vi "MDAQ_ReverseCalibration.vi"(8 "MDU Velocity":dbl, 9 "MDAQ Calibration":dbl, 10 "Main Cluster in":T1, 11 "Status_Cluster In":T2 {"GATESTOP" format="%04x"; "GATESTRT" format="%04x"; "AMPLITUDE" format="%04x"; "M_CYCLES" format="%04x"; "N_CYCLES" format="%04x"; "STEP" format="%04x"; "BASE" format="%04x"; "CHAN" format="%04x"}) -> (1 "Scaler":dbl, 2 "output cluster":T1)   [LabVIEW 2021]
uses:
  <vilib>/Analysis/NI_AALPro.lvlib
  Status_Cluster.ctl
  GUI_Def.ctl
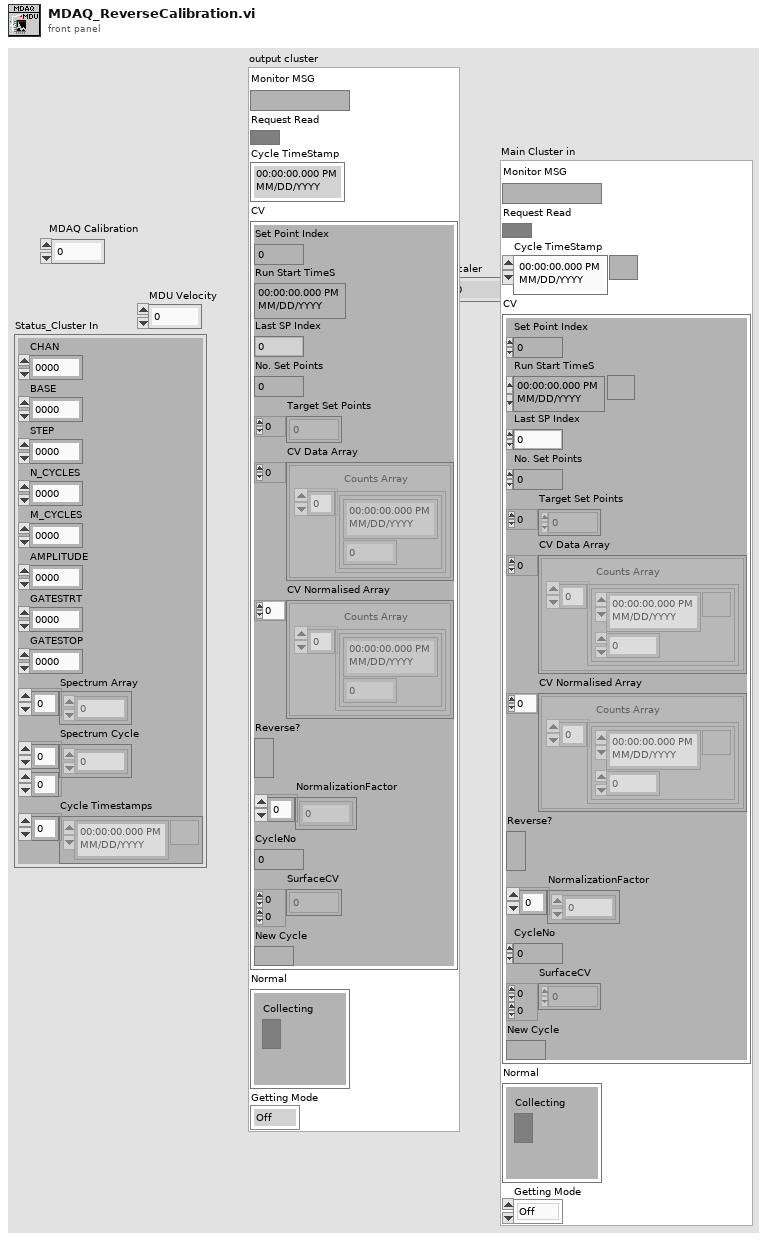
[diagram p1: front panel]
types:
  T1 = typedef "GUI_Def.ctl" = cluster{"Monitor MSG":string, "Request Read":bool, "Cycle TimeStamp":timestamp, "CV":cluster{"Set Point Index":u32, "Run Start TimeS":timestamp, "Last SP Index":u32, "No. Set Points":u32, "Target Set Points":dbl[], "CV Data Array":cluster{"Counts Array":cluster{timestamp, i32}[]}[], "CV Normalised Array":cluster{"Counts Array":cluster{timestamp, dbl}[]}[], "Reverse?":bool, "NormalizationFactor":i32[], "CycleNo":i32, "SurfaceCV":dbl[][], "New Cycle":bool}, "Normal":cluster{"Collecting":bool}, "Getting Mode":enum16{"Off", "Normal", "CV"}}
  T2 = typedef "Status_Cluster.ctl" = cluster{"CHAN":u32, "BASE":u32, "STEP":u32, "N_CYCLES":u32, "M_CYCLES":u32, "AMPLITUDE":u32, "GATESTRT":u32, "GATESTOP":u32, "Spectrum Array":u32[], "Spectrum Cycle":u32[][], "Cycle Timestamps":timestamp[]}
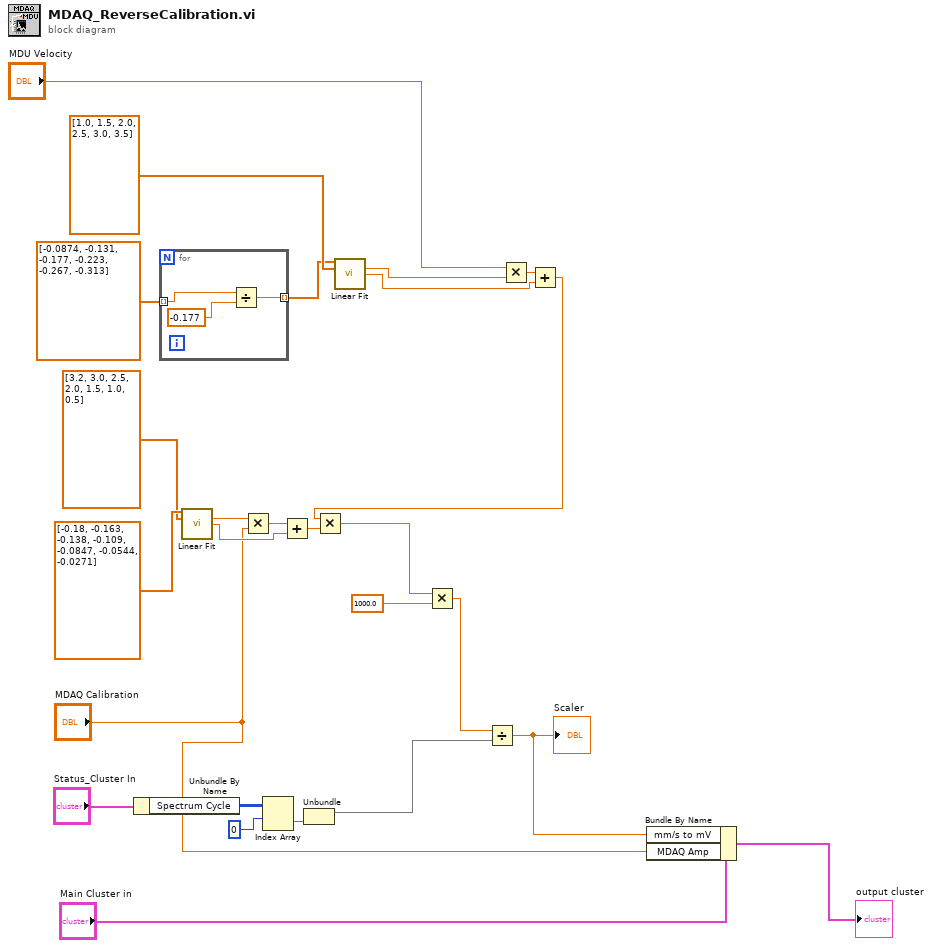
[diagram p0: block diagram]
diagram:
  n1 = Unbundle By Name("Status_Cluster In") -> ("Spectrum Cycle"=w9:u32[][])
  n2 = for {
    tunnel: dbl[] [-0.0874, -0.131, -0.177, -0.223, -0.267, -0.313] -> [w29] mode=indexing
    tunnel: [w27] -> w24 mode=indexing
    n3 = Divide(x=w29, y=-0.177) -> (x/y=w27:dbl)
  }
  n4 = call <vilib>:"Linear Fit.vi"("Y"=dbl[] [-0.18, -0.163, -0.138, -0.109, -0.0847, -0.0544, -0.0271], "X"=dbl[] [3.2, 3.0, 2.5, 2.0, 1.5, 1.0, 0.5]) -> ("slope"=w17:dbl, "intercept"=w15:dbl)  [unwired: 9 in, 3 out]
  n5 = Multiply(x=w17, y="MDAQ Calibration") -> (x*y=w16:dbl)
  n6 = Index Array(array=w9, index (row)=0 ("index")) -> (element=w7:u32[])  [unwired: 1 in]
  n7 = Add(x=w16, y=w15) -> (x+y=w14:dbl)
  n8 = Unbundle(w7) -> (w5)  [unwired: 1 out]
  n9 = call <vilib>:"Linear Fit.vi"("Y"=w24, "X"=dbl[] [1.0, 1.5, 2.0, 2.5, 3.0, 3.5]) -> ("slope"=w23:dbl, "intercept"=w20:dbl)  [unwired: 9 in, 3 out]
  n10 = Multiply(x="MDU Velocity", y=w23) -> (x*y=w21:dbl)
  n11 = Add(x=w21, y=w20) -> (x+y=w13:dbl)
  n12 = Multiply(x=w13, y=w14) -> (x*y=w12:dbl)
  n13 = Multiply(x=w12, y=1000.0) -> (x*y=w6:dbl)
  n14 = Divide(x=w6, y=w5) -> (x/y=w3:dbl)
  "Scaler" <- w3
  n15 = Bundle By Name(cluster="Main Cluster in", "mm/s to mV"=w3, "MDAQ Amp"="MDAQ Calibration") -> (→"output cluster":T1)
